vi "readTag.vi"(8 "error in (no error)":errorcluster, 11 "PLC in":refnum<class "PLC.lvclass">) -> (0 "error out":errorcluster, 3 "PLC out":refnum<class "PLC.lvclass">)   [LabVIEW 2020, in "PLC.lvclass"]
uses:
  PLC.lvclass
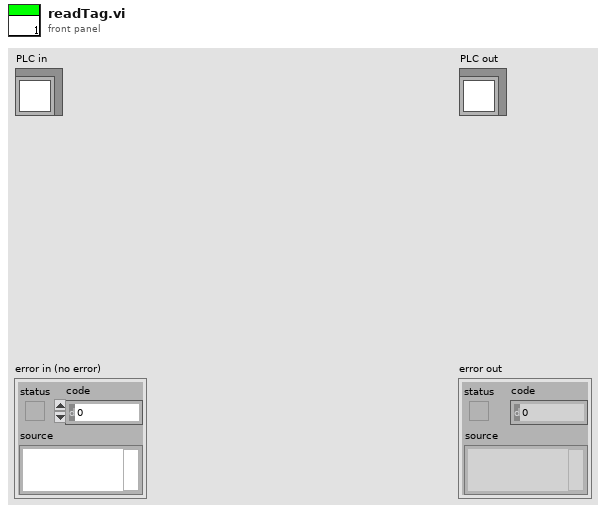
[diagram p1: front panel]
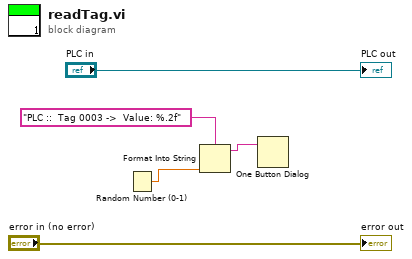
[diagram p0: block diagram]
diagram:
  n1 = Random Number (0-1)() -> (number: 0 to 1=w3:dbl)
  n2 = Format Into String(format string="PLC ::  Tag 0003 ->  Value: %.2f" ("message"), w3) -> (resulting string=w2:string)  [unwired: 2 in, 1 out]
  n3 = One Button Dialog(message=w2) -> ()  [unwired: 1 in, 1 out]
  "error out" <- "error in (no error)"
  "PLC out" <- "PLC in"
